vi "Get Start + End Distances.vi"(8 "error in (no error)":errorcluster, 11 "Test Cluster":T1) -> (0 "error out":errorcluster, 2 "End Distance":dbl, 3 "Start Distance":dbl)   [LabVIEW 2024]
uses:
  Controls/Test Cluster.ctl
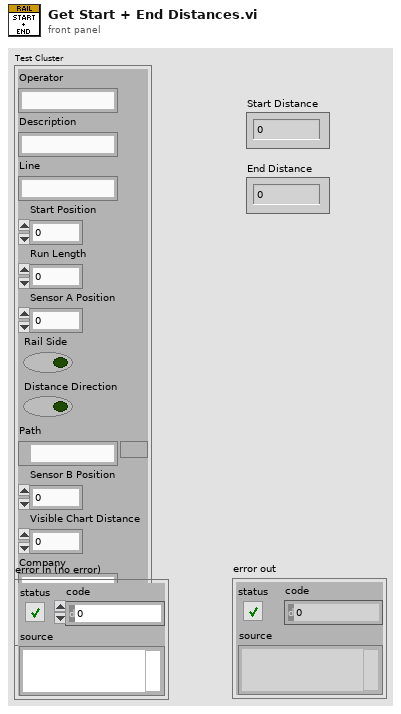
[diagram p1: front panel]
types:
  T1 = typedef "Test Cluster.ctl" = cluster{"Operator":string, "Description":string, "Line":string, "Start Position":dbl, "Run Length":dbl, "Sensor A Position":dbl, "Rail Side":bool, "Distance Direction":bool, "Path":path, "Sensor B Position":dbl, "Visible Chart Distance":dbl, "Company":string, "Ref Profile":string}
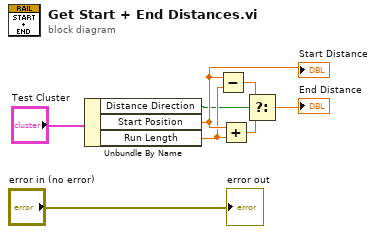
[diagram p0: block diagram]
diagram:
  n1 = Unbundle By Name("Test Cluster") -> ("Distance Direction"=w3:bool, "Start Position"=w8:dbl, "Run Length"=w6:dbl)
  "Start Distance" <- w8
  n2 = Subtract(x=w8, y=w6) -> (x-y=w4:dbl)
  n3 = Add(x=w8, y=w6) -> (x+y=w5:dbl)
  n4 = Select(t=w4, s=w3, f=w5) -> (s? t:f=→"End Distance":dbl)
  "error out" <- "error in (no error)"
